vi "Test_Commands.vi"() -> ()   [LabVIEW 2017, in "WordManipulationTests.lvlib"]
uses:
  WordManipulationTests.lvlib
  Utilities/Controlword_Commands.ctl
  Utilities/WordManipulationLibrary.lvlib
panel:
  out "ControlWord":u16[](array[numeric]) format="%08b"
  out "Initial Command":T1[](array[typedef])
  out "WordToCommand":T1[](array[typedef])
  out "Equal?":bool[](array[boolean])
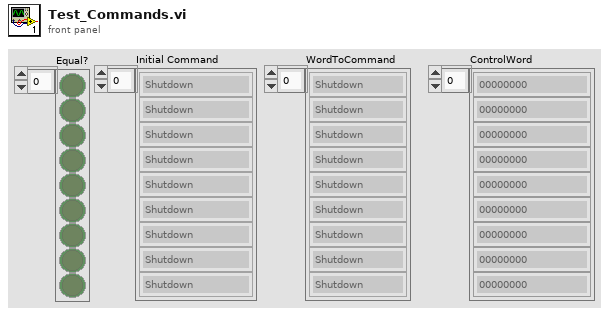
[diagram p1: front panel]
types:
  T1 = typedef "WordManipulationLibrary.lvlib/Controlword_Commands.ctl" = enum16{"Shutdown", "Switch On", "Disable Voltage", "Quick Stop", "Disable Op", "Enable Op", "Fault Reset", "Error"}
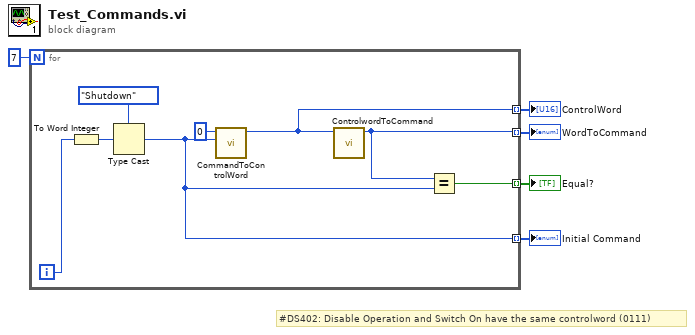
[diagram p0: block diagram]
diagram:
  # "#DS402: Disable Operation and Switch On have the same controlword (0111)"
  n1 = for {
    N: 7 -> [_]
    tunnel: [w11] -> w4 mode=indexing
    tunnel: [w10] -> w3 mode=indexing
    tunnel: [w9] -> w2 mode=indexing
    tunnel: [w6] -> w1 mode=indexing
    i -> [w8]
    n2 = To Word Integer(number=w8) -> (16bit integer=w7:i16)
    n3 = Type Cast(type=Controlword_Commands."Shutdown" ("Device Control Command"), x=w7) -> (*(type *) &x=w9:T1)
    n4 = call "CommandToControlWord.vi"("Device Control Command"=w9, "ControlWord In"=u16 0) -> ("ControlWord Out"=w6:u16)  [unwired: 9 in]
    n5 = call "ControlwordToCommand.vi"("Data_In"=w6) -> ("Device Control Command"=w10:T1)  [unwired: 10 in]
    n6 = Equal?(x=w10, y=w9) -> (x = y?=w11:bool)
  }
  "Equal?" <- w4
  "WordToCommand" <- w3
  "Initial Command" <- w2
  "ControlWord" <- w1
